vi "Read Credentials.vi"(8 "error in (no error)":errorcluster, 11 "AWS Core in":refnum<class "HTTP Request.lvclass">) -> (0 "error out":errorcluster, 2 "Credentials":T1, 3 "AWS Core out":refnum<class "HTTP Request.lvclass">)   [LabVIEW 2015, in "NI_AWS_Core.lvlib" / "HTTP Request.lvclass"]
uses:
  HTTP Request.lvclass
  AWS Credentials.ctl
  HTTP Request.lvclass/HTTP Request.ctl
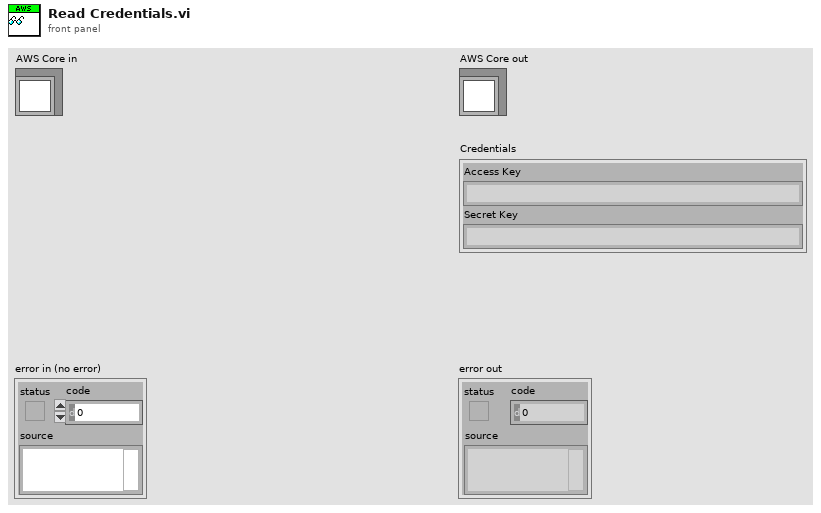
[diagram p1: front panel]
types:
  T1 = typedef "NI_AWS_Core.lvlib/HTTP Request.lvclass/AWS Credentials.ctl" = cluster{"Access Key":string, "Secret Key":string}
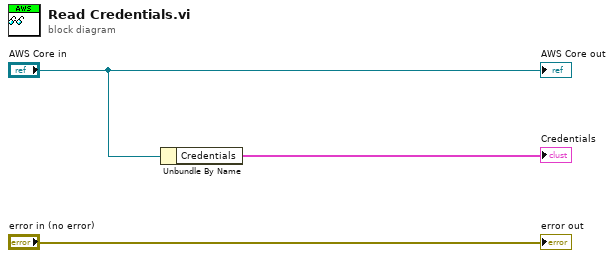
[diagram p0: block diagram]
diagram:
  n1 = Unbundle By Name("AWS Core in") -> ("Credentials"=→"Credentials":T1)
  "error out" <- "error in (no error)"
  "AWS Core out" <- "AWS Core in"
